vi "NULLcharacterKILLER.vi"(1 "String":string="\u00007\u0000.\u00005\u00005\u00008\u0000E\u0000+\u00000\u00005\u0000", 2 "Enum":enum16{"First", "Second"}(ring)) -> (0 "string":string)   [LabVIEW 2019]
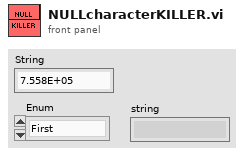
[diagram p1: front panel]
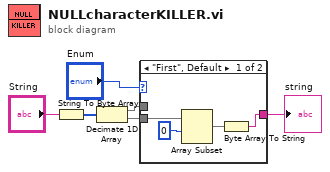
[diagram p0: block diagram]
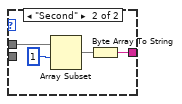
[diagram p2: hidden frame]
diagram:
  n1 = String To Byte Array(string="String") -> (unsigned byte array=w6:u8[])
  n2 = Decimate 1D Array(w6) -> (w2:u8[], w5:u8[])
  n3 = case shown="\"First\", Default" "Enum" {
    tunnel: [w9 w13] -> w1
    tunnel: w5 -> [w8 _]
    tunnel: w2 -> [_ w12]
    frame "First", Default {
      n4 = Array Subset(array=w8, index=0) -> (w10:u8[])  [unwired: 1 in]
      n5 = Byte Array To String(unsigned byte array=w10) -> (string=w9:string)
    }
    frame "Second" {
      n6 = Array Subset(array=w12, index=1) -> (w14:u8[])  [unwired: 1 in]
      n7 = Byte Array To String(unsigned byte array=w14) -> (string=w13:string)
    }
  }
  "string" <- w1
